vi "summing_the_money (SubVI).vi"(11 "Money":T1) -> (3 "Numeric":dbl)   [LabVIEW 2020]
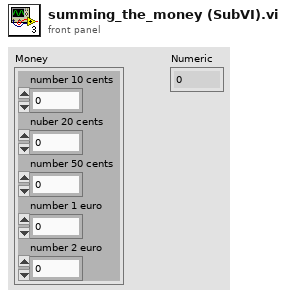
[diagram p1: front panel]
types:
  T1 = cluster{"number 10 cents":dbl, "nuber 20 cents":dbl, "number 50 cents":dbl, "number 1 euro":dbl, "number 2 euro":dbl}
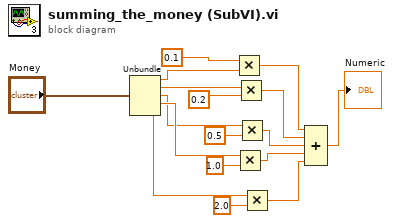
[diagram p0: block diagram]
diagram:
  n1 = Unbundle("Money") -> ("number 10 cents"=w2:dbl, "nuber 20 cents"=w4:dbl, "number 50 cents"=w6:dbl, "number 1 euro"=w8:dbl, "number 2 euro"=w10:dbl)
  n2 = Multiply(x=0.1, y=w2) -> (x*y=w13:dbl)
  n3 = Multiply(x=w8, y=1.0) -> (x*y=w16:dbl)
  n4 = Multiply(x=w4, y=0.2) -> (x*y=w14:dbl)
  n5 = Multiply(x=w6, y=0.5) -> (x*y=w15:dbl)
  n6 = Multiply(x=w10, y=2.0) -> (x*y=w17:dbl)
  n7 = Compound Arithmetic op=ADD(w13, w14, w15, w16, w17) -> (→"Numeric":dbl)
